vi "wd_repalceInIndex (WFM).vi"(6 "data type":T7, 7 "WFM":waveform(dbl), 8 "error in (no error)":errorcluster, 9 "value index":u64, 10 "channel index":u32, 11 "meta in":T1={"TargetFile"=path "", "StreamMode"=enum."File", "Append?"=FALSE, "ChunkSize"=0, "TimeColumnMode"=enum."Empty", "TimestampFormat"="", "AbsoluteTime?"=FALSE, "FileAttribute "={"Creator"="", "Title"="", "SheetName"=""}, "Column"=[], "FileRef"=refnum, "MemoryRef"=[], "RecordInfo"=[], " ChannelPreviousInfo"=[], "ChannelFirstRecord"=[], "PredefinedFormattedValueLength"=20, "DiskTemplate"={"XMLRef"=[refnum, refnum, refnum, refnum, refnum, refnum], "ZipPath"=path "", "MetaFile"={"Ref"=refnum, "NextRow"=0, "NextPosition"=0, "Block"=[]}, "TempFolder"=path ""}}) -> (0 "error out":errorcluster, 3 "meta out":T1={"TargetFile"=path "", "StreamMode"=enum."File", "Append?"=FALSE, "ChunkSize"=0, "TimeColumnMode"=enum."Empty", "TimestampFormat"="", "AbsoluteTime?"=FALSE, "FileAttribute "={"Creator"="", "Title"="", "SheetName"=""}, "Column"=[], "FileRef"=refnum, "MemoryRef"=[], "RecordInfo"=[], " ChannelPreviousInfo"=[], "ChannelFirstRecord"=[], "PredefinedFormattedValueLength"=20, "DiskTemplate"={"XMLRef"=[refnum, refnum, refnum, refnum, refnum, refnum], "ZipPath"=path "", "MetaFile"={"Ref"=refnum, "NextRow"=0, "NextPosition"=0, "Block"=[]}, "TempFolder"=path ""}})   [LabVIEW 2020, in "NI_ExcelFile.lvlib"]
uses:
  <vilib>/express/express shared/NI_ExcelFile/NI_ExcelFile.lvlib
  <vilib>/express/express shared/NI_ExcelFile/Ctrls/DataType.ctl
  <vilib>/express/express shared/NI_ExcelFile/Ctrls/MainData.ctl
  <vilib>/express/express shared/NI_ExcelFile/Ctrls/StreamMode.ctl
  <vilib>/express/express shared/NI_ExcelFile/Ctrls/TimeColumnMode.ctl
  <vilib>/express/express shared/NI_ExcelFile/Ctrls/FileAttribute.ctl
  <vilib>/express/express shared/NI_ExcelFile/Ctrls/Columns.ctl
  <vilib>/express/express shared/NI_ExcelFile/Ctrls/ColumnInfo.ctl
  <vilib>/express/express shared/NI_ExcelFile/Ctrls/wd_recordInfo.ctl
  <vilib>/express/express shared/NI_ExcelFile/Ctrls/disk_TemplateFile.ctl
  <vilib>/express/express shared/NI_ExcelFile/Ctrls/meta_file.ctl
  <vilib>/express/express shared/NI_ExcelFile/Ctrls/meta_Block.ctl
  <vilib>/express/express shared/NI_ExcelFile/Ctrls/meta_BlockType.ctl
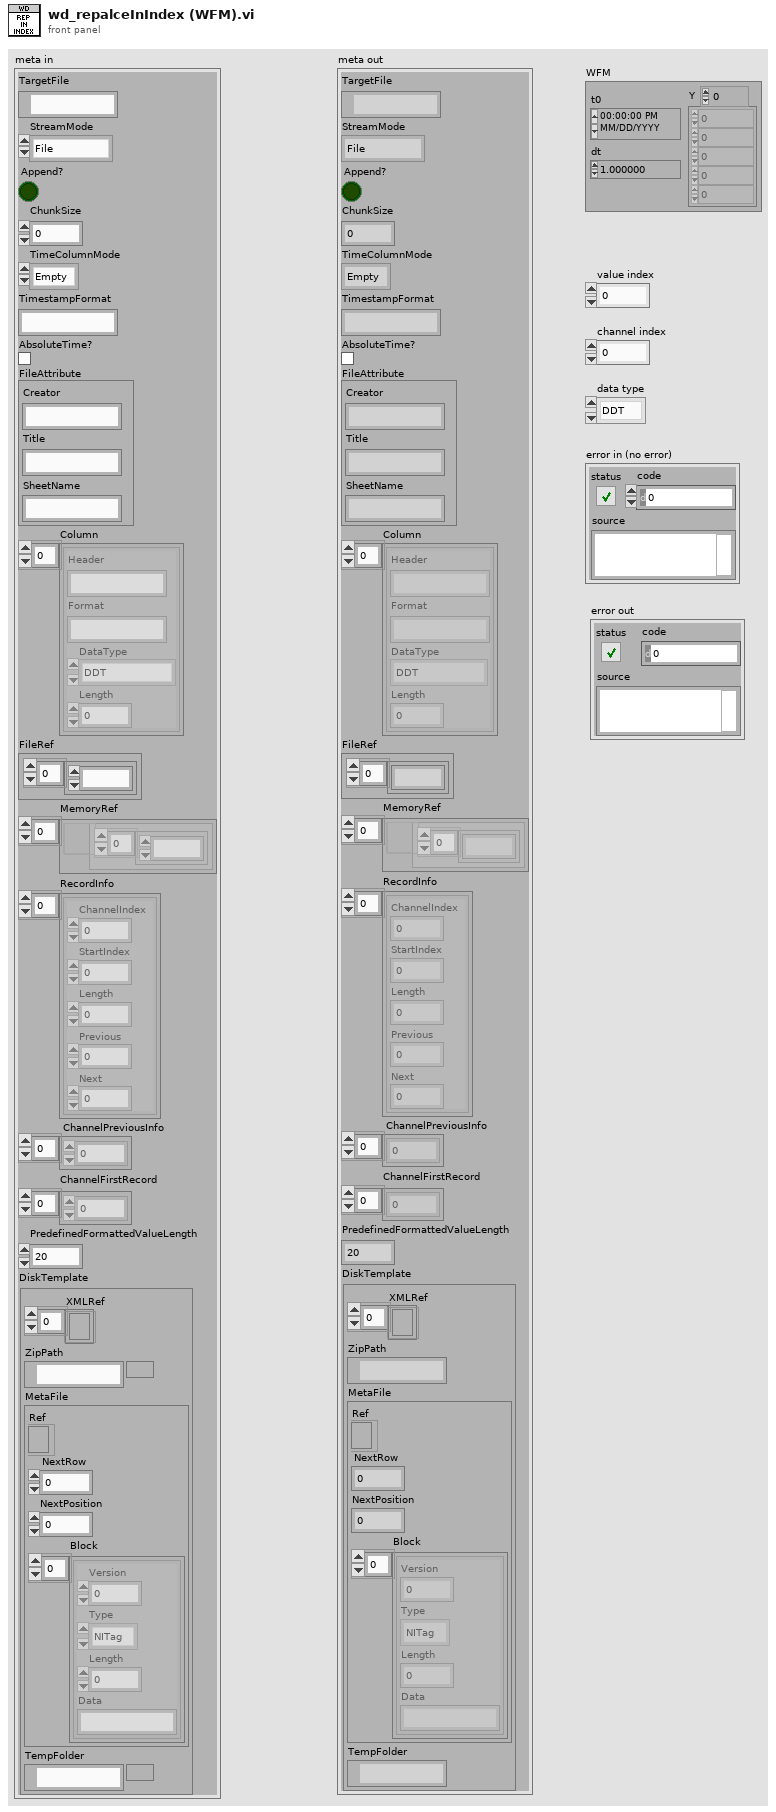
[diagram p1: front panel]
types:
  T1 = typedef "NI_ExcelFile.lvlib/MainData.ctl" = cluster{"TargetFile":path, "StreamMode":T2, "Append?":bool, "ChunkSize":u64, "TimeColumnMode":T3, "TimestampFormat":string, "AbsoluteTime?":bool, "FileAttribute ":T4, "Column":T5, "FileRef":refnum<k1>, "MemoryRef":refnum<data-value>[], "RecordInfo":T8[], " ChannelPreviousInfo":u32[], "ChannelFirstRecord":u32[], "PredefinedFormattedValueLength":i64, "DiskTemplate":T9}
  T2 = typedef "NI_ExcelFile.lvlib/StreamMode.ctl" = enum16{"File", "Memory"}
  T3 = typedef "NI_ExcelFile.lvlib/TimeColumnMode.ctl" = enum16{"Empty", "OnePerCh", "One"}
  T4 = typedef "NI_ExcelFile.lvlib/FileAttribute.ctl" = cluster{"Creator":string, "Title":string, "SheetName":string}
  T5 = typedef "NI_ExcelFile.lvlib/Columns.ctl" = T6[]
  T6 = typedef "NI_ExcelFile.lvlib/ColumnInfo.ctl" = cluster{"Header":string, "Format":string, "DataType":T7, "Length":u64}
  T7 = typedef "NI_ExcelFile.lvlib/DataType.ctl" = enum16{"DDT", "WFM", "Array of STR", "Array of DBL", "Array of I8", "Array of I16", "Array of I32", "Array of I64", "Array of SGL", "Array of U8", "Array of U16", "Array of U32", "Array of U64", "Array of Time"}
  T8 = typedef "NI_ExcelFile.lvlib/wd_recordInfo.ctl" = cluster{"ChannelIndex":u32, "StartIndex":u64, "Length":u64, "Previous":i32, "Next":i32}
  T9 = typedef "NI_ExcelFile.lvlib/disk_TemplateFile.ctl" = cluster{"XMLRef":refnum<file>[], "ZipPath":path, "MetaFile":T10, "TempFolder":path}
  T10 = typedef "NI_ExcelFile.lvlib/meta_file.ctl" = cluster{"Ref":refnum<file>, "NextRow":i32, "NextPosition":i64, "Block":T11[]}
  T11 = typedef "NI_ExcelFile.lvlib/meta_Block.ctl" = cluster{"Version":u16, "Type":T12, "Length":i32, "Data":string}
  T12 = typedef "NI_ExcelFile.lvlib/meta_BlockType.ctl" = enum16{"NITag", "File", "Column"}
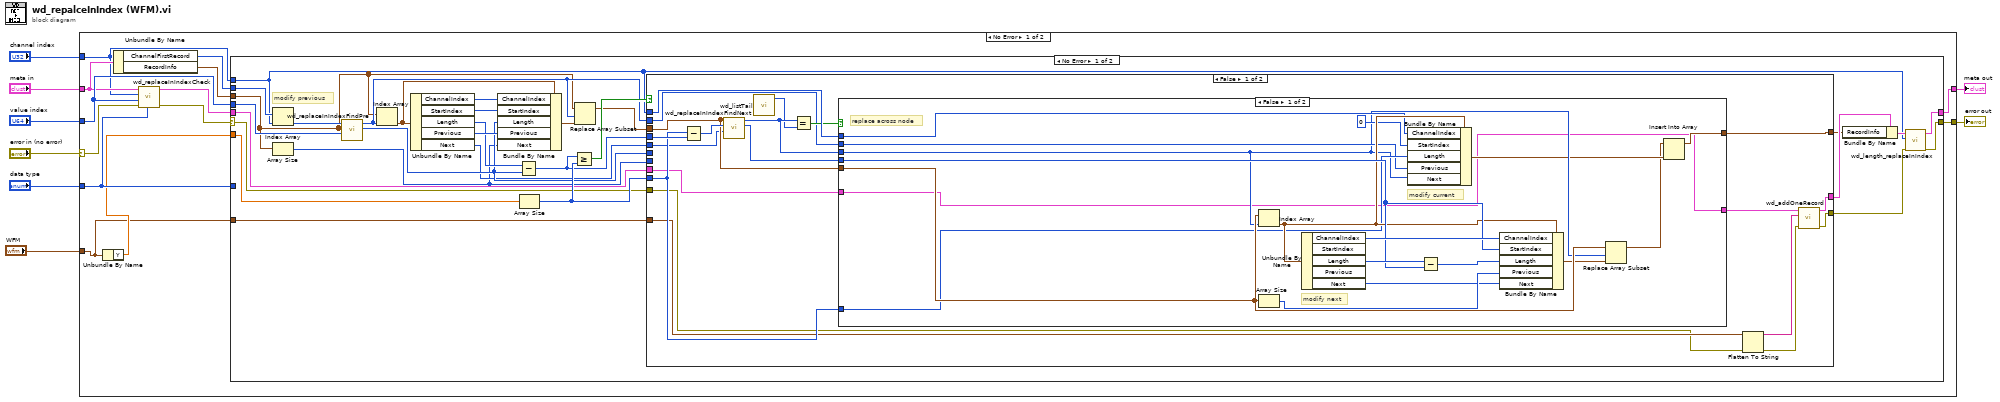
[diagram p0: block diagram]
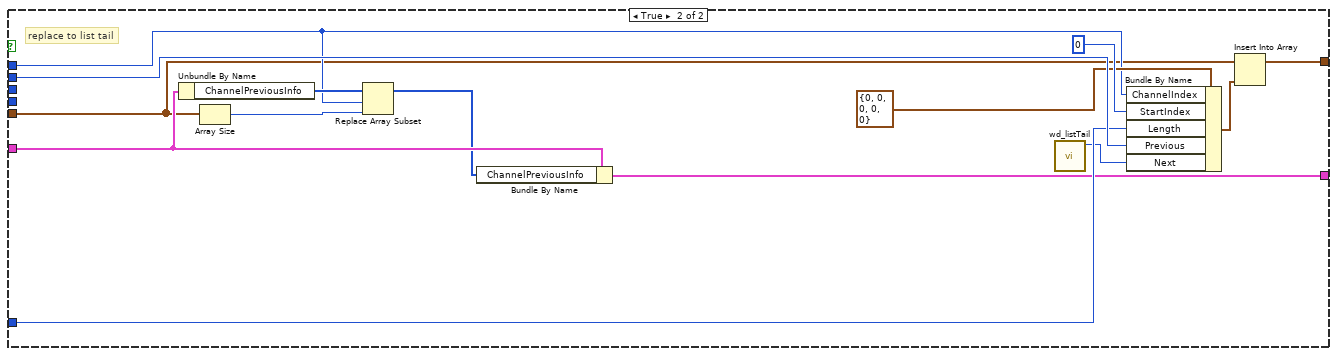
[diagram p2: hidden frame]
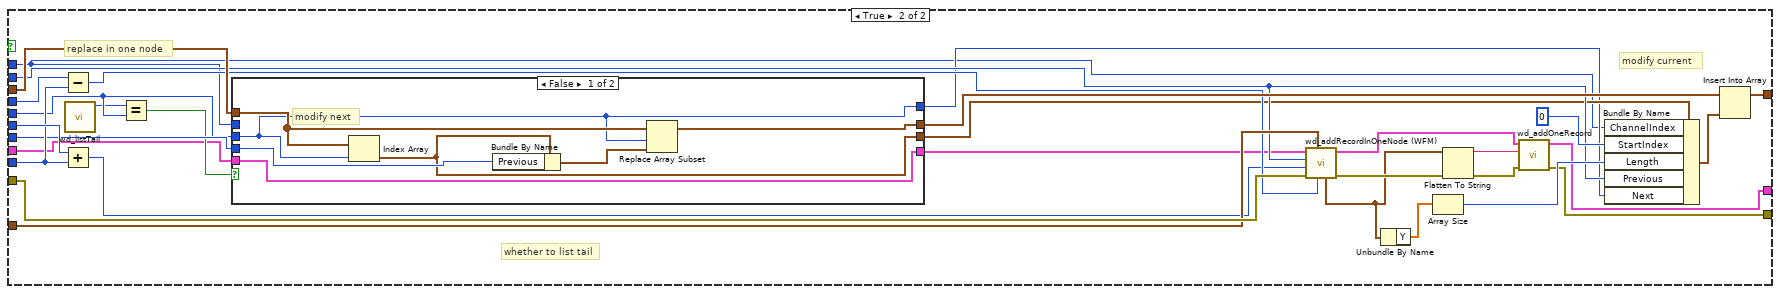
[diagram p3: hidden frame]
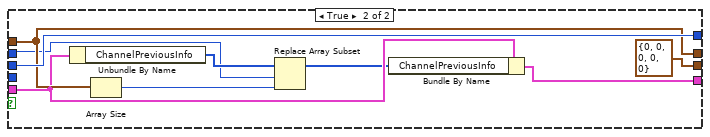
[diagram p4: hidden frame]
diagram:
  n1 = case shown="No Error" "error in (no error)" {
    selector: "error in (no error)" -> [w12 w153]
    tunnel: "channel index" -> [w15 _]
    tunnel: "meta in" -> [w16 w152]
    tunnel: "value index" -> [w19 _]
    tunnel: [w21 w153] -> w2
    tunnel: [w20 w152] -> w5
    tunnel: "data type" -> [w13 _]
    tunnel: "WFM" -> [w9 _]
    frame No Error {
      n2 = Unbundle By Name(w9) -> ("Y"=w10:dbl[])
      n3 = Unbundle By Name(w16) -> ("ChannelFirstRecord"=w18:u32[], "RecordInfo"=w17:T8[])
      n4 = call <vilib>:"wd_replaceInIndexCheck.vi"("data type"=w13, "error in (no error)"=w12, "value index"=w19, "channel index"=w15, "meta in"=w16) -> ("error out"=w11:errorcluster, "meta out"=w14:T1)  [unwired: 5 in]
      n5 = case shown="No Error" w11 {
        selector: w11 -> [w25 w150]
        tunnel: w14 -> [w35 w151]
        tunnel: w10 -> [w34 _]
        tunnel: [w30 w151] -> w20
        tunnel: [w23 w150] -> w21
        tunnel: w15 -> [w26 _]
        tunnel: w19 -> [w49 _]
        tunnel: w18 -> [w32 _]
        tunnel: w17 -> [w31 _]
        tunnel: w13 -> [_ _]
        tunnel: w9 -> [w22 _]
        frame No Error {
          # "modify previous"
          n6 = Index Array(array=w32, index=w26) -> (element=w50:u32)
          n7 = Array Size(array=w31) -> (size(s)=w36:i32)
          n8 = call <vilib>:"wd_replaceInIndexFindPre.vi"("value index"=w49, "RecordInfo"=w31, "node start index"=w50) -> ("value index out"=w40:u64, "pre node index"=w41:i32)  [unwired: 7 in]
          n9 = Index Array(array=w31, index=w41) -> (element=w33:T8)
          n10 = Unbundle By Name(w33) -> ("ChannelIndex"=w48:u32, "StartIndex"=w47:u64, "Length"=w44:u64, "Previous"=w46:i32, "Next"=w38:i32)
          n11 = Bundle By Name(cluster=w33, "ChannelIndex"=w48, "StartIndex"=w47, "Length"=w40, "Previous"=w46, "Next"=w36) -> (w45:T8)
          n12 = Subtract(x=w44, y=w40) -> (x-y=w39:u64)
          n13 = Array Size(array=w34) -> (size(s)=w42:i32)
          n14 = Greater Or Equal?(x=w39, y=w42) -> (x >= y?=w43:bool)
          n15 = Replace Array Subset(array=w31, new element=w45, index=w41) -> (w37:T8[])
          n16 = case shown="False" w43 {
            tunnel: w26 -> [w66 w106]
            tunnel: w42 -> [w67 w130]
            tunnel: w41 -> [w53 w116]
            tunnel: w35 -> [w60 w108]
            tunnel: w22 -> [w57 w120]
            tunnel: w40 -> [_ w132]
            tunnel: w39 -> [w70 w131]
            tunnel: w38 -> [w52 w111]
            tunnel: w37 -> [w63 w125]
            tunnel: [w68 w126] -> w27
            tunnel: w36 -> [_ w129]
            tunnel: [w58 w121] -> w29
            tunnel: w25 -> [w55 w123]
            tunnel: [w61 w122] -> w24
            frame False {
              n17 = Subtract(x=w67, y=w70) -> (x-y=w69:u64)
              n18 = call <vilib>:"wd_replaceInIndexFindNext.vi"("Next in"=w52, "LengthIn"=w69, "RecordInfo"=w63) -> ("LengthOut"=w64:u64, "Next out"=w62:i32)  [unwired: 7 in]
              n19 = call <vilib>:"wd_listTail.vi"() -> ("list tail"=w51:i32)  [unwired: 11 in]
              n20 = Equal?(x=w62, y=w51) -> (x = y?=w65:bool)
              n21 = case shown="False" w65 {
                tunnel: w63 -> [w82 w90]
                tunnel: w62 -> [w75 _]
                tunnel: w64 -> [w85 _]
                tunnel: [w72 w92] -> w68
                tunnel: w66 -> [w79 w91]
                tunnel: w67 -> [w77 w98]
                tunnel: w53 -> [w76 w101]
                tunnel: w60 -> [w71 w96]
                tunnel: [w71 w94] -> w59
                frame False {
                  # "replace across node"
                  # "modify current"
                  # "modify next"
                  n22 = Index Array(array=w82, index=w75) -> (element=w80:T8)
                  n23 = Array Size(array=w82) -> (size(s)=w84:i32)
                  n24 = Unbundle By Name(w80) -> ("ChannelIndex"=w88:u32, "Length"=w86:u64, "Next"=w83:i32)  [unwired: 2 out]
                  n25 = Bundle By Name(cluster=w80, "ChannelIndex"=w79, "StartIndex"=u64 0 ("Start Index"), "Length"=w77, "Previous"=w76, "Next"=w75) -> (w74:T8)
                  n26 = Subtract(x=w86, y=w85) -> (x-y=w87:u64)
                  n27 = Bundle By Name(cluster=w80, "ChannelIndex"=w88, "StartIndex"=w85, "Length"=w87, "Previous"=w84, "Next"=w83) -> (w81:T8)
                  n28 = Replace Array Subset(array=w82, new element=w81, index=w75) -> (w73:T8[])
                  n29 = Insert Into Array(array=w73, new element=w74) -> (w72:T8[])  [unwired: 1 in]
                }
                frame True {
                  # "replace to list tail"
                  n30 = Unbundle By Name(w96) -> ("ChannelPreviousInfo"=w99:u32[])
                  n31 = Array Size(array=w90) -> (size(s)=w97:i32)
                  n32 = Replace Array Subset(array=w99, new element=w97, index=w91) -> (w95:u32[])
                  n33 = Bundle By Name(cluster=w96, "ChannelPreviousInfo"=w95) -> (w94:T1)
                  n34 = call <vilib>:"wd_listTail.vi"() -> ("list tail"=w89:i32)  [unwired: 11 in]
                  n35 = Bundle By Name(cluster=T8 {"ChannelIndex"=0, "StartIndex"=0, "Length"=0, "Previous"=0, "Next"=0} ("output cluster"), "ChannelIndex"=w91, "StartIndex"=u64 0 ("Start Index"), "Length"=w98, "Previous"=w101, "Next"=w89) -> (w100:T8)
                  n36 = Insert Into Array(array=w90, new element=w100) -> (w92:T8[])  [unwired: 1 in]
                }
              }
              n37 = Flatten To String(anything=w57, error in (no error)=w55) -> (data string=w56:string, error out=w54:errorcluster)  [unwired: 2 in, 1 out]
              n38 = call <vilib>:"wd_addOneRecord.vi"("error in (no error)"=w54, "data"=w56, "meta in"=w59) -> ("error out"=w61:errorcluster, "meta out"=w58:T1)  [unwired: 7 in]
            }
            frame True {
              # "whether to list tail"
              # "replace in one node"
              # "modify current"
              n39 = Subtract(x=w131, y=w130) -> (x-y=w118:u64)
              n40 = Add(x=w132, y=w130) -> (x+y=w117:u64)
              n41 = call <vilib>:"wd_listTail.vi"() -> ("list tail"=w105:i32)  [unwired: 11 in]
              n42 = Equal?(x=w105, y=w111) -> (x = y?=w110:bool)
              n43 = case shown="False" w110 {
                tunnel: w129 -> [w140 _]
                tunnel: [w138 w147] -> w128
                tunnel: w125 -> [w137 w147]
                tunnel: [w136 T8 {"ChannelIndex"=0, "StartIndex"=0, "Length"=0, "Previous"=0, "Next"=0} ("RecordInfo")] -> w115
                tunnel: w111 -> [w135 w148]
                tunnel: [w135 w148] -> w109
                tunnel: w108 -> [w134 w143]
                tunnel: [w134 w141] -> w107
                tunnel: w106 -> [_ w145]
                frame False {
                  # "modify next"
                  n44 = Index Array(array=w137, index=w135) -> (element=w136:T8)
                  n45 = Bundle By Name(cluster=w136, "Previous"=w140) -> (w139:T8)
                  n46 = Replace Array Subset(array=w137, new element=w139, index=w135) -> (w138:T8[])
                }
                frame True {
                  n47 = Unbundle By Name(w143) -> ("ChannelPreviousInfo"=w146:u32[])
                  n48 = Array Size(array=w147) -> (size(s)=w144:i32)
                  n49 = Replace Array Subset(array=w146, new element=w144, index=w145) -> (w142:u32[])
                  n50 = Bundle By Name(cluster=w143, "ChannelPreviousInfo"=w142) -> (w141:T1)
                }
              }
              n51 = call <vilib>:"wd_addRecordInOneNode (WFM).vi"("length"=w118, "waveform"=w120, "error in (no error)"=w123, "start"=w117, "datalog postion"=w116, "meta in"=w107) -> ("error out"=w113:errorcluster, "meta out"=w119:T1, "waveform out"=w104:waveform(dbl))  [unwired: 3 in]
              n52 = Unbundle By Name(w104) -> ("Y"=w103:dbl[])
              n53 = Array Size(array=w103) -> (size(s)=w124:i32)
              n54 = Flatten To String(anything=w104, error in (no error)=w113) -> (data string=w114:string, error out=w112:errorcluster)  [unwired: 2 in, 1 out]
              n55 = call <vilib>:"wd_addOneRecord.vi"("error in (no error)"=w112, "data"=w114, "meta in"=w119) -> ("error out"=w122:errorcluster, "meta out"=w121:T1)  [unwired: 7 in]
              n56 = Bundle By Name(cluster=w115, "ChannelIndex"=w106, "StartIndex"=u64 0 ("Start Index"), "Length"=w124, "Previous"=w116, "Next"=w109) -> (w127:T8)
              n57 = Insert Into Array(array=w128, new element=w127) -> (w126:T8[])  [unwired: 1 in]
            }
          }
          n58 = Bundle By Name(cluster=w29, "RecordInfo"=w27) -> (w28:T1)
          n59 = call <vilib>:"wd_length_replaceInIndex.vi"("error in (no error)"=w24, "channel index"=w26, "meta in"=w28) -> ("error out"=w23:errorcluster, "meta out"=w30:T1)  [unwired: 7 in]
        }
        frame Error {
        }
      }
    }
    frame Error {
    }
  }
  "meta out" <- w5
  "error out" <- w2
